vi "Register gRPC Messages.vi"(8 "error in (no error)":errorcluster, 11 "gRPC ID":T1) -> (0 "error out":errorcluster, 3 "gRPC ID Out":T1)   [LabVIEW 2021, in "dcvmDPI_AD7606B_client.lvlib"]
uses:
  dcvmDPI_AD7606B_client.lvlib
  <vilib>/gRPC/LabVIEW gRPC Library/Shared/grpcId.ctl
  <vilib>/gRPC/LabVIEW gRPC Library/Server API/typeDefs/Message Metadata.ctl
  <vilib>/gRPC/LabVIEW gRPC Library/Server API/typeDefs/Message Element Metadata.ctl
  <vilib>/gRPC/LabVIEW gRPC Library/Server API/typeDefs/Message Element Type.ctl
  <vilib>/gRPC/LabVIEW gRPC Library/grpc-lvsupport-release.lvlib
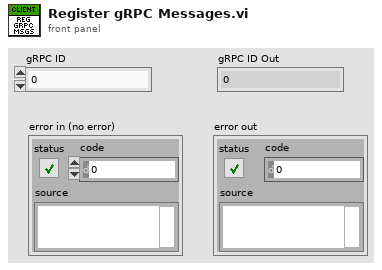
[diagram p1: front panel]
types:
  T1 = typedef "grpc-lvsupport-release.lvlib/grpcId.ctl" = u64
  T2 = typedef "grpc-lvsupport-release.lvlib/Message Metadata.ctl" = cluster{"Version":i32, "Name":string, "Type Url":string, "Elements":T3[]}
  T3 = typedef "grpc-lvsupport-release.lvlib/Message Element Metadata.ctl" = cluster{"Embedded Message Name":string, "Protobuf Index":i32, "MessageElementType":T4, "Repeated":bool}
  T4 = typedef "grpc-lvsupport-release.lvlib/Message Element Type.ctl" = enum32{"Int32Value", "FloatValue", "DoubleValue", "BoolValue", "StringValue", "MessageValue", "Int64Value", "UInt32Value", "UInt64Value", "EnumValue", "Bytes", "Fixed64", "Fixed32", "SFixed64", "SFixed32", "SInt64", "SInt32"}
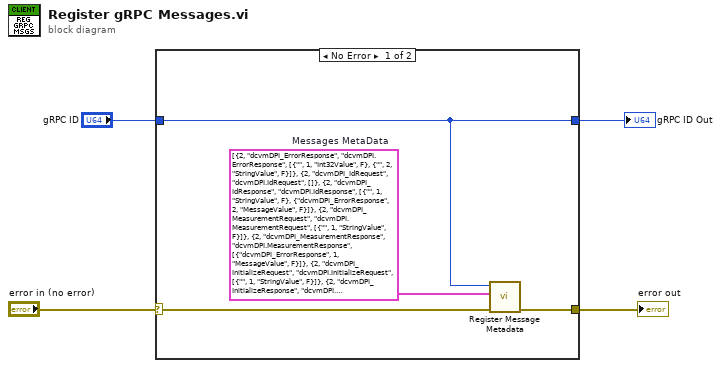
[diagram p0: block diagram]
diagram:
  n1 = case shown="No Error" "error in (no error)" {
    selector: "error in (no error)" -> [w6 w10]
    tunnel: [w5 w9] -> w1
    tunnel: [w8 w10] -> w4
    tunnel: "gRPC ID" -> [w5 w9]
    frame No Error {
      w7 = T2[] [{"Version"=2, "Name"="dcvmDPI_ErrorResponse", "Type Url"="dcvmDPI.ErrorResponse", "Elements"=[{"Embedded Message Name"="", "Protobuf Index"=1, "MessageElementType"=enum."Int32Value", "Repeated"=FALSE}, {"Embedded Message Name"="", "Protobuf Index"=2, "MessageElementType"=enum."StringValue", "Repeated"=FALSE}]}, {"Version"=2, "Name"="dcvmDPI_IdRequest", "Type Url"="dcvmDPI.IdRequest", "Elements"=[]}, {"Version"=2, "Name"="dcvmDPI_IdResponse", "Type Url"="dcvmDPI.IdResponse", "Elements"=[{"Embedded Message Name"="", "Protobuf Index"=1, "MessageElementType"=enum."StringValue", "Repeated"=FALSE}, {"Embedded Message Name"="dcvmDPI_ErrorResponse", "Protobuf Index"=2, "MessageElementType"=enum."MessageValue", "Repeated"=FALSE}]}, {"Version"=2, "Name"="dcvmDPI_MeasurementRequest", "Type Url"="dcvmDPI.MeasurementRequest", "Elements"=[{"Embedded Message Name"="", "Protobuf Index"=1, "MessageElementType"=enum."StringValue", "Repeated"=FALSE}]}, {"Version"=2, "Name"="dcvmDPI_MeasurementResponse", "Type Url"="dcvmDPI.MeasurementResponse", "Elements"=[{"Embedded Message Name"="dcvmDPI_ErrorResponse", "Protobuf Index"=1, "MessageElementType"=enum."MessageValue", "Repeated"=FALSE}]}, {"Version"=2, "Name"="dcvmDPI_InitializeRequest", "Type Url"="dcvmDPI.InitializeRequest", "Elements"=[{"Embedded Message Name"="", "Protobuf Index"=1, "MessageElementType"=enum."StringValue", "Repeated"=FALSE}]}, {"Version"=2, "Name"="dcvmDPI_InitializeResponse", "Type Url"="dcvmDPI.InitializeResponse", "Elements"=[{"Embedded Message Name"="dcvmDPI_ErrorResponse", "Protobuf Index"=1, "MessageElementType"=enum."MessageValue", "Repeated"=FALSE}]}, {"Version"=2, "Name"="dcvmDPI_ConfigureRequest", "Type Url"="dcvmDPI.ConfigureRequest", "Elements"=[{"Embedded Message Name"="", "Protobuf Index"=1, "MessageElementType"=enum."UInt32Value", "Repeated"=FALSE}, {"Embedded Message Name"="", "Protobuf Index"=2, "MessageElementType"=enum."DoubleValue", "Repeated"=FALSE}, {"Embedded Message Name"="", "Protobuf Index"=3, "MessageElementType"=enum."Int32Value", "Repeated"=FALSE}]}, {"Version"=2, "Name"="dcvmDPI_ConfigureResponse", "Type Url"="dcvmDPI.ConfigureResponse", "Elements"=[{"Embedded Message Name"="dcvmDPI_ErrorResponse", "Protobuf Index"=1, "MessageElementType"=enum."MessageValue", "Repeated"=FALSE}]}, {"Version"=2, "Name"="dcvmDPI_InitiateRequest", "Type Url"="dcvmDPI.InitiateRequest", "Elements"=[]}, {"Version"=2, "Name"="dcvmDPI_InitiateResponse", "Type Url"="dcvmDPI.InitiateResponse", "Elements"=[{"Embedded Message Name"="dcvmDPI_ErrorResponse", "Protobuf Index"=1, "MessageElementType"=enum."MessageValue", "Repeated"=FALSE}]}, {"Version"=2, "Name"="dcvmDPI_AcquireRequest", "Type Url"="dcvmDPI.AcquireRequest", "Elements"=[{"Embedded Message Name"="", "Protobuf Index"=1, "MessageElementType"=enum."UInt32Value", "Repeated"=FALSE}, {"Embedded Message Name"="", "Protobuf Index"=2, "MessageElementType"=enum."Int32Value", "Repeated"=FALSE}]}, {"Version"=2, "Name"="dcvmDPI_AcquireResponse", "Type Url"="dcvmDPI.AcquireResponse", "Elements"=[{"Embedded Message Name"="", "Protobuf Index"=1, "MessageElementType"=enum."UInt32Value", "Repeated"=TRUE}, {"Embedded Message Name"="dcvmDPI_ErrorResponse", "Protobuf Index"=2, "MessageElementType"=enum."MessageValue", "Repeated"=FALSE}]}, {"Version"=2, "Name"="dcvmDPI_CloseRequest", "Type Url"="dcvmDPI.CloseRequest", "Elements"=[]}, {"Version"=2, "Name"="dcvmDPI_CloseResponse", "Type Url"="dcvmDPI.CloseResponse", "Elements"=[{"Embedded Message Name"="dcvmDPI_ErrorResponse", "Protobuf Index"=1, "MessageElementType"=enum."MessageValue", "Repeated"=FALSE}]}]  # Messages MetaData
      n2 = call <vilib>:"Register Message Metadata.vi"("error in"=w6, "Messages"=w7, "gRPCid in"=w5) -> ("error out"=w8:errorcluster)  [unwired: 7 in, 1 out]
    }
    frame Error {
    }
  }
  "error out" <- w4
  "gRPC ID Out" <- w1
